vi "State Change.vi"(4 "User Parameter":variant, 5 "Event Data":cluster{"sender":refnum<k24>, "e":refnum<k24>}, 6 "Control Ref":refnum<k24>, 7 "Event Common Data":T1) -> ()   [LabVIEW 2022 SP3]
uses:
  C:/Software Repos/shared components/SECSGEM/DotNet20EqApp/GemEqApp/SecsPort.dll
  Software Repos/shared components/SECSGEM/DotNet20EqApp/GemEqApp/SecsPort.dll
panel:
  out "newvalue":string
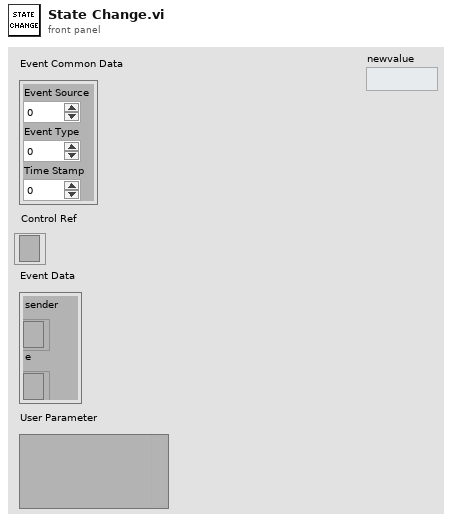
[diagram p1: front panel]
types:
  T1 = cluster{"Event Source":i32, "Event Type":u32, "Time Stamp":u32}
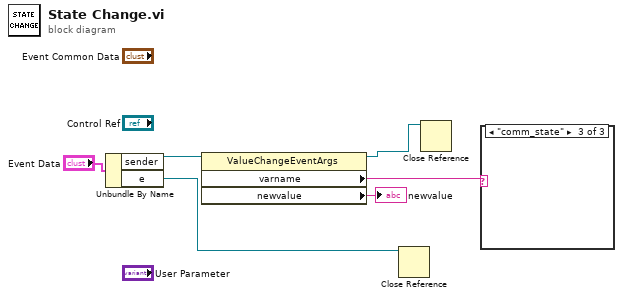
[diagram p0: block diagram]
diagram:
  n1 = Unbundle By Name("Event Data") -> ("e"=w2:refnum<k24>)  [unwired: 1 out]
  n2 = property class="ValueChangeEventArgs"(reference=w2) -> (reference out=w3:refnum<k24>, "varname"=w4:string, "newvalue"=→"newvalue":string)  [unwired: 1 in, 1 out]
  n3 = Close Reference(reference=w2) -> ()  [unwired: 1 in, 1 out]
  n4 = Close Reference(reference=w3) -> ()  [unwired: 1 in, 1 out]
  n5 = case shown="\"comm_state\"" w4 {
    frame "control_state" {
    }
    frame Default {
    }
    frame "comm_state" {
    }
  }
